vi "Tab Page Enable Disable.vi"() -> ()   [LabVIEW 2022 SP3]
panel:
  in  "Thermometer":dbl(slide) scale=0.0..100.0
  in  "Tab Control":enum32{"Page 1", "Page 2", "Page 3"}(tab)
  out "Boolean 2":bool
  in  "Boolean":bool
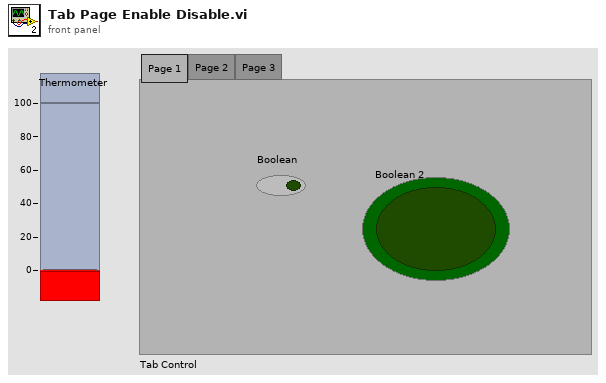
[diagram p1: front panel]
types:
  T1 = enum8{"Enabled", "Disabled", "Disabled and Grayed Out"}
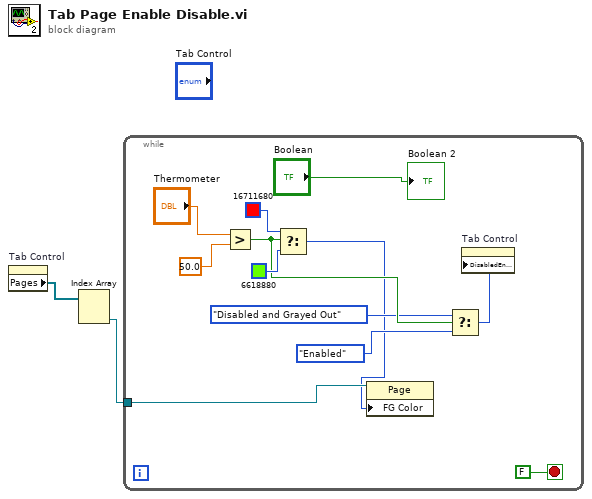
[diagram p0: block diagram]
diagram:
  n1 = property on="Tab Control" class="TabCtl (strict)"() -> ("Pages"=w2:refnum<vi>[])  [unwired: 2 in, 2 out]
  n2 = Index Array(array=w2) -> (element #2=w1:refnum<vi>)  [unwired: 2 in, 1 out]
  n3 = while {
    tunnel: w1 -> [w4]
    stop <- FALSE stop-if-true
    n4 = Greater?(x="Thermometer", y=50.0) -> (0:w9:bool)
    n5 = Select(t=u32 16711680, s=w9, f=u32 6618880) -> (s? t:f=w3:u32)
    n6 = property class="Page"(reference=w4, "FG Color"=w3) -> ()  [unwired: 1 in, 2 out]
    n7 = Select(t=T1."Disabled and Grayed Out" ("Disabled"), s=w9, f=T1."Enabled" ("Disabled")) -> (s? t:f=w6:T1)
    n8 = property on="Tab Control" class="TabCtl (strict)"("DisabledEnum"=w6) -> ()  [unwired: 2 in, 2 out]
    "Boolean 2" <- "Boolean"
  }
